vi "Bernoulli Noise (obs 90).vi"(2 "seed":i32=-1, 3 "ones probability":dbl=0.5 format="%0.2f", 4 "samples":i32=128) -> (0 "error":i32, 1 "bernoulli noise":u8[](array[numeric]))   [LabVIEW 2010, in "NI_AALBase.lvlib"]
doc: "The Bernoulli Noise VI was rewritten in LabVIEW 2009. Replace this VI with a Bernoulli Noise VI from the <B>Functions</B> palette to use the new functionality.\n\nGenerates a pseudorandom pattern of ones and zeroes. LabVIEW computes each element of <B>bernoulli noise</B> as if flipping a coin weighted by <B>ones probability</B>."
uses:
  NI_AALBase.lvlib
panel:
  # "Bernoulli Noise"
  # "This VI is obsolete !!!\nYou should replace this VI in your diagram with the Bernoulli Noise VI."
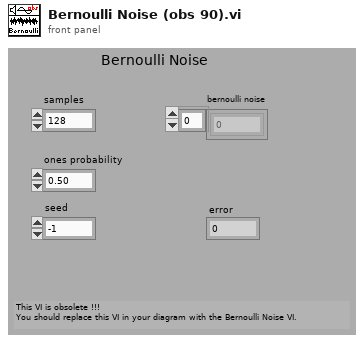
[diagram p1: front panel]
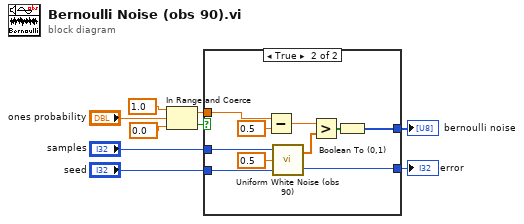
[diagram p0: block diagram]
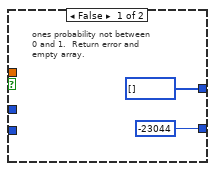
[diagram p2: hidden frame]
diagram:
  n1 = In Range and Coerce(upper limit=1.0, x="ones probability", lower limit=0.0) -> (coerced(x)=w2:dbl, In Range?=w3:bool)
  n2 = case shown="True" w3 {
    tunnel: [-23044 ("error") w21] -> w9
    tunnel: "seed" -> [_ w20]
    tunnel: "samples" -> [_ w19]
    tunnel: [i16[] [] w16] -> w6
    tunnel: w2 -> [_ w12]
    frame False {
      # "ones probability not between \n0 and 1.  Return error and \nempty array."
    }
    frame True {
      n3 = Subtract(x=w12, y=0.5) -> (x-y=w15:dbl)
      n4 = call "Uniform White Noise (obs 90).vi"("seed"=w20, "amplitude"=0.5, "samples"=w19) -> ("error"=w21:i32, "uniform white noise"=w13:dbl[])
      n5 = Greater?(x=w15, y=w13) -> (0:w17:bool[])
      n6 = Boolean To (0,1)(Boolean=w17) -> (0, 1=w16:i16[])
    }
  }
  "error" <- w9
  "bernoulli noise" <- w6
